vi "pf_List_Properties.vi"(8 "error in (no error)":errorcluster, 11 "IMAQ Session in":refnum<k11>) -> (0 "error out":errorcluster, 2 "Properties List":T1[](array[typedef]), 3 "IMAQ Session out":refnum<k11>)   [LabVIEW 2025, in "Photonfocus_Toolkit.lvlib"]
doc: "Scans the camera for properties and outputs a properties list (array of properties clusters)."
uses:
  Photonfocus_Toolkit.lvlib
  _Private/Controls/pf_Property_Info.ctl
  _Private/Controls/pf_Property_Type.ctl
  _Private/Controls/pf_Property_Flag.ctl
  _Private/Controls/pf_Camera_ctrl_mngr_action.ctl
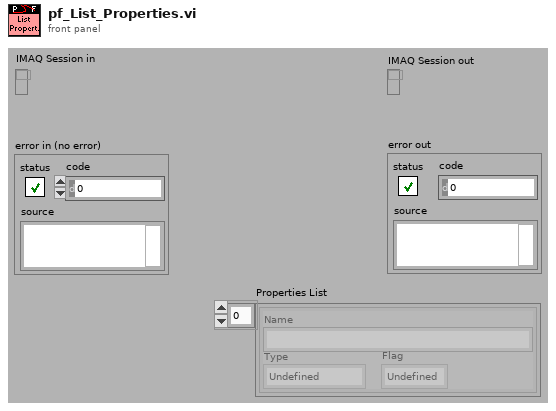
[diagram p1: front panel]
types:
  T1 = typedef "Photonfocus_Toolkit.lvlib/pf_Property_Info.ctl" = cluster{"Name":string, "Type":T2, "Flag":T3}
  T2 = typedef "Photonfocus_Toolkit.lvlib/pf_Property_Type.ctl" = enum16{"Undefined", "PF_ROOT", "PF_INT", "PF_FLOAT", "PF_BOOL", "PF_MODE", "PF_REGISTER", "PF_STRING", "PF_BUFFER", "PF_STRUCT", "PF_ARRAY", "PF_COMMAND", "PF_EVENT"}
  T3 = typedef "Photonfocus_Toolkit.lvlib/pf_Property_Flag.ctl" = enum16{"Undefined", "RO", "WO", "RW"}
  T4 = typedef "Photonfocus_Toolkit.lvlib/pf_Camera_ctrl_mngr_action.ctl" = enum16{"Create", "Destroy", "Set", "Get"}
  T5 = typedef "Photonfocus_Toolkit.lvlib/pf_Property_Cluster.ctl" = cluster{"Name":string, "Type":T2, "Float.Min":sgl, "Float.Max":sgl, "Float.Value":sgl, "Int.Min":u32, "Int.Max":u32, "Int.Value":u32, "String.Value":string, "MODE.Values":string[], "MODE.Index":i32, "Flag":T3}
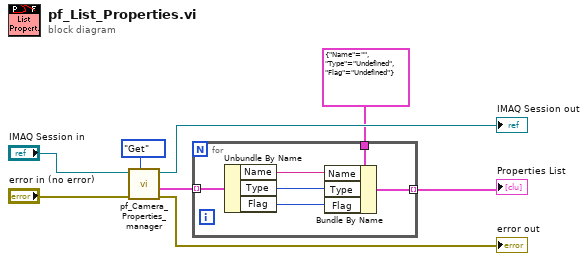
[diagram p0: block diagram]
diagram:
  n1 = call "pf_Camera_Properties_manager.vi"("Action"=pf_Camera_ctrl_mngr_action."Get", "error in (no error)"="error in (no error)", "IMAQ Session in"="IMAQ Session in") -> ("error out"=→"error out":errorcluster, "Properties Array out"=w5:T5[], "IMAQ Session out"=→"IMAQ Session out":refnum<k11>)  [unwired: 2 in, 4 out]
  n2 = for {
    tunnel: w5 -> [w14] mode=indexing
    tunnel: T1 {"Name"="", "Type"=enum."Undefined", "Flag"=enum."Undefined"} ("Property Info") -> [w13]
    tunnel: [w9] -> w1 mode=indexing
    n3 = Unbundle By Name(w14) -> ("Name"=w12:string, "Type"=w11:T2, "Flag"=w10:T3)
    n4 = Bundle By Name(cluster=w13, "Name"=w12, "Type"=w11, "Flag"=w10) -> (w9:T1)
  }
  "Properties List" <- w1
